vi "AlazarSetBWLimit.vi"(3 "error in (no error)":errorcluster, 4 "Flag":u32(ring) items=["Disable Limit", "Enable Limit"], 5 "Channel":u32(ring)=1 items=["A"=1, "B"=2, "C"=4, "D"=8], 6 "Handle":u32) -> (0 "error out":errorcluster, 1 "Return Code":u32, 2 "Handle":u32)   [LabVIEW 2018]
doc: "Control bandwidth of an input channel."
uses:
  ATSApi.dll
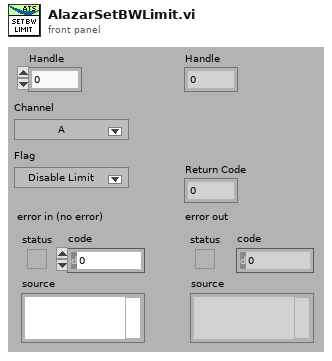
[diagram p1: front panel]
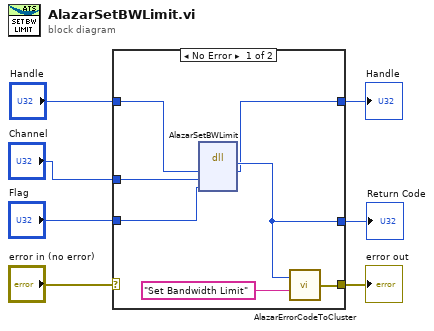
[diagram p0: block diagram]
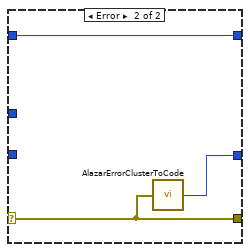
[diagram p2: hidden frame]
diagram:
  n1 = case shown="No Error" "error in (no error)" {
    selector: "error in (no error)" -> [_ w17]
    tunnel: [w11 w17] -> w6
    tunnel: [w13 w16] -> w5
    tunnel: "Handle" -> [w14 w15]
    tunnel: [w10 w15] -> w3
    tunnel: "Channel" -> [w9 _]
    tunnel: "Flag" -> [w8 _]
    frame No Error {
      n2 = dll-call lib="ATSApi.dll" fn="AlazarSetBWLimit"("handle"=w14, "channelId"=w9, "flag"=w8) -> (w13:u32, "handle"=w10:u32)  [unwired: 5 in, 2 out]
      n3 = call "AlazarErrorCodeToCluster.vi"("Message"="Set Bandwidth Limit", "Error Code"=w13) -> ("error out"=w11:errorcluster)
    }
    frame Error {
      n4 = call "AlazarErrorClusterToCode.vi"("error in (no error)"=w17) -> ("Error Code"=w16:u32)
    }
  }
  "Handle" <- w3
  "error out" <- w6
  "Return Code" <- w5
